vi "EncoderRateToRPM.vi"(10 "Enum":enum16{"DirectMag", "Through Bore", "Mag"}(ring), 11 "EncoderRate":dbl) -> (2 "RPM":dbl, 3 "RPS":dbl)   [LabVIEW 2019]
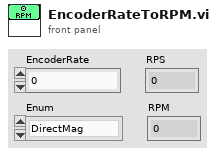
[diagram p1: front panel]
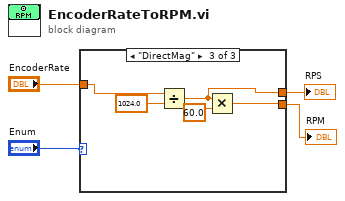
[diagram p0: block diagram]
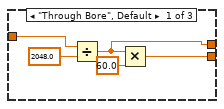
[diagram p2: hidden frame]
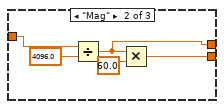
[diagram p3: hidden frame]
diagram:
  n1 = case shown="\"DirectMag\"" "Enum" {
    tunnel: "EncoderRate" -> [w7 w14 w17]
    tunnel: [w6 w11 w16] -> w2
    tunnel: [w5 w10 w15] -> w1
    frame "Through Bore", Default {
      n2 = Divide(x=w7, y=2048.0) -> (x/y=w6:dbl)
      n3 = Multiply(x=w6, y=60.0) -> (x*y=w5:dbl)
    }
    frame "Mag" {
      n4 = Divide(x=w14, y=4096.0) -> (x/y=w11:dbl)
      n5 = Multiply(x=w11, y=60.0) -> (x*y=w10:dbl)
    }
    frame "DirectMag" {
      n6 = Divide(x=w17, y=1024.0) -> (x/y=w16:dbl)
      n7 = Multiply(x=w16, y=60.0) -> (x*y=w15:dbl)
    }
  }
  "RPM" <- w1
  "RPS" <- w2
